vi "working with signals.vi"() -> ()   [LabVIEW 2018]
uses:
  <vilib>/Analysis/3filter.llb/Filter Passband Type.ctl
  <vilib>/Analysis/2dsp.llb/Power Spectrum (DBL).vi
  <vilib>/Analysis/3filter.llb/Butterworth Filter (DBL).vi
  <vilib>/Analysis/NI_AALBase.lvlib
  <vilib>/Analysis/NI_AALPro.lvlib
panel:
  out "Waveform Graph 4":dbl[](graph)
  out "Waveform Graph 2":dbl[][](graph)
  in  "filter type":T1
  in  "order":i32=2
  out "Waveform Graph":dbl[](graph)
  in  "Knob":dbl(knob) scale=0.0..10.0
  in  "width":i32=1
  in  "delay":i32
  in  "samples":i32=128
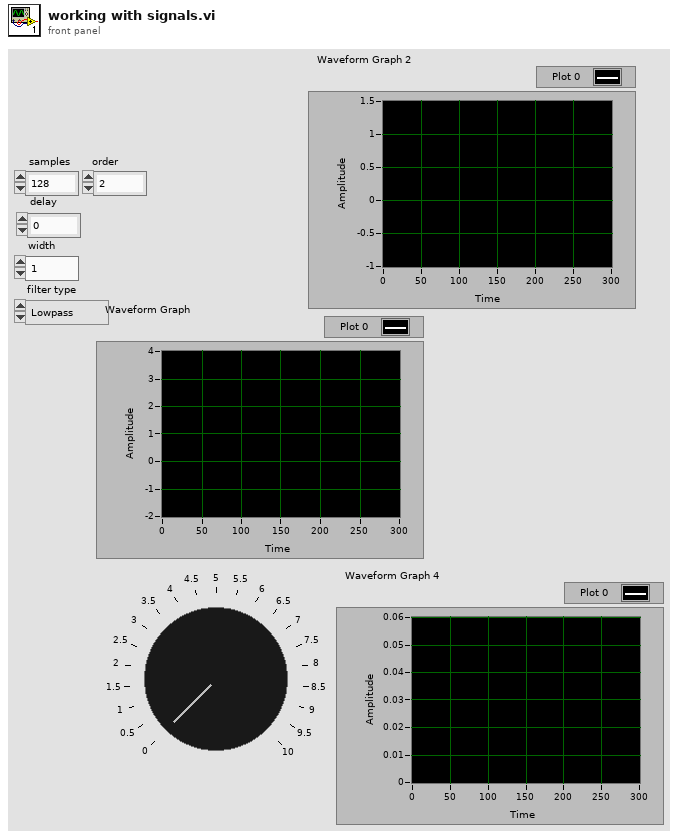
[diagram p1: front panel]
types:
  T1 = typedef "NI_AALBase.lvlib/Filter Passband Type.ctl" = enum32{"Lowpass", "Highpass", "Bandpass", "Bandstop"}
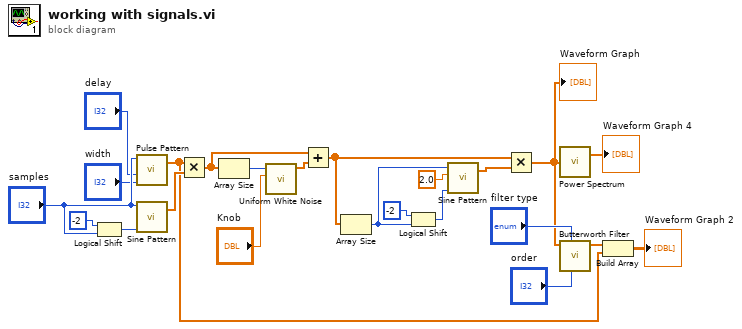
[diagram p0: block diagram]
diagram:
  n1 = Logical Shift(y=i16 -2, x="samples") -> (x << y=w23:i32)
  n2 = call <vilib>:"Pulse Pattern.vi"("width"="width", "delay"="delay", "samples"="samples") -> ("Pulse Pattern"=w5:dbl[])  [unwired: 1 in, 1 out]
  n3 = call <vilib>:"Sine Pattern.vi"("cycles"=w23, "samples"="samples") -> ("Sinusoidal Pattern"=w18:dbl[])  [unwired: 2 in, 1 out]
  n4 = Multiply(x=w5, y=w18) -> (x*y=w3:dbl[])
  n5 = Array Size(array=w3) -> (size(s)=w17:i32)
  n6 = call <vilib>:"Uniform White Noise.vi"("amplitude"="Knob", "samples"=w17) -> ("uniform white noise"=w15:dbl[])  [unwired: 8 in, 1 out]
  n7 = Add(x=w3, y=w15) -> (x+y=w10:dbl[])
  n8 = Array Size(array=w10) -> (size(s)=w9:i32)
  n9 = Logical Shift(y=i16 -2, x=w9) -> (x << y=w14:i32)
  n10 = call <vilib>:"Sine Pattern.vi"("cycles"=w14, "amplitude"=2.0, "samples"=w9) -> ("Sinusoidal Pattern"=w11:dbl[])  [unwired: 1 in, 1 out]
  n11 = Multiply(x=w10, y=w11) -> (x*y=w1:dbl[])
  "Waveform Graph" <- w1
  n12 = call-poly <vilib>:"Power Spectrum.vi"("X"=w1) -> ("Power Spectrum"=→"Waveform Graph 4":dbl[])  [unwired: 1 out]
  n13 = call-poly <vilib>:"Butterworth Filter.vi"("order"="order", "filter type"="filter type", "X"=w1) -> ("Filtered X"=w6:dbl[])  [unwired: 5 in, 1 out]
  n14 = Build Array(w6, w5) -> (→"Waveform Graph 2":dbl[][])
